vi "ENTHALdll.vi"(8 "error in (no error)":errorcluster, 9 "z":dbl[](array[numeric]), 10 "D":dbl, 11 "t":dbl) -> (0 "error out":errorcluster, 3 "h":dbl)   [LabVIEW 2021]
doc: "subroutine ENTHALdll(t, d, z, h)\n\nCompute enthalpy as a function of temperature, density, and\ncomposition using core functions (Helmholtz free energy and ideal\ngas integrals)\n\nBased on derivations in Younglove & McLinden, JPCRD 23 #5, 1994,\nequations A7, A18, A19\n\nINPUTS:\nt -- temperature [K]\nD -- molar density [mol/L]\nz -- composition [array of mol frac]\n\nOUTPUT:\nh -- enthalpy [J/mol]"
uses:
  REFPROP.dll
panel:
  # "REFPROP-ENTHALdll.vi"
  # "void  ENTHALdll(double *t, double *D, double *z, double *h);"
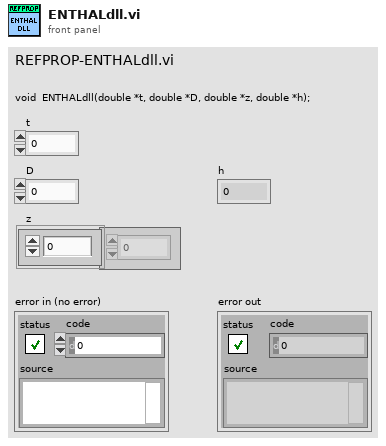
[diagram p1: front panel]
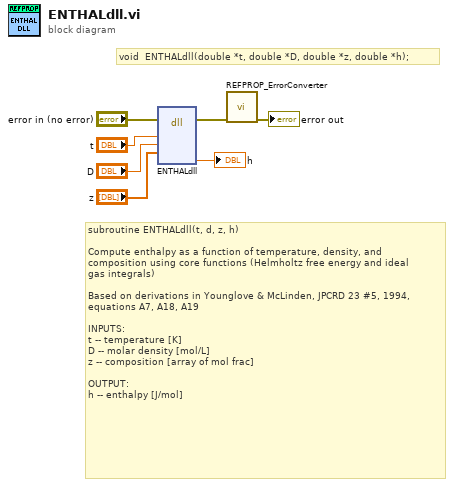
[diagram p0: block diagram]
diagram:
  # "void  ENTHALdll(double *t, double *D, double *z, double *h);"
  # "subroutine ENTHALdll(t, d, z, h)\n\nCompute enthalpy as a function of temperature, density, and\ncomposition using core functions (Helmholtz free energy and ideal\ngas integrals)\n\nBased on derivations in Younglove & McLinden, JPCRD 23 #5, 1994,\nequations A7, A18, A19\n\nINPUTS:\nt -- temperature [K]\nD -- molar density [mol/L]\nz -- composition [array of mol frac]\n\nOUTPUT:\nh -- enthalpy [J/mol]"
  n1 = dll-call lib="C:/Users/lauria/OneDrive - National Institute of Standards and Technology (NIST)/LabVIEW Projects/7 REFPROP/REFPROP-wrappers-master/REFPROP-wrappers-master/wrappers/Labview/REFPROP/REFPROP.*" fn="ENTHALdll"(error in="error in (no error)", "t"="t", "D"="D", "z"="z") -> (error out=w3:errorcluster, "h"=→"h":dbl)  [unwired: 7 in, 1 out]
  n2 = call "REFPROP_ErrorConverter.vi"("error in (no error)"=w3) -> ("error out"=→"error out":errorcluster)  [unwired: 10 in]
